vi "generate path.vi"(8 "Config":T1={"Path"={"Spacing"=2608.0, "Smooth Weight"=0.3, "Tolerance"=0.01}, "Kinematics"={"Max Vel"=2000.0, "Max Accel"=200.0, "Curvature Const"=2.0}}, 11 "Waypoints":dbl[][](array[numeric])=[[0.0, 0.0], [100.0, 15648.0], [10342.0, 25000.0]]) -> (0 "Target Velocities":dbl[](array[numeric])=[2000.0, 2000.0, 2000.0, 2000.0, 2000.0, 2000.0, 2000.0, 2000.0, 2000.0, 2000.0, 2000.0, 2000.0, 711.0227082060944, 0.0], 1 "Curvatures":dbl[](array[numeric])=[0.0, 3.4302286185049717e-08, 1.4910129056131163e-07, 6.219521538995594e-07, 2.6949817858486045e-06, 1.4154000940659975e-05, 0.00023495395525552563, 0.00023525971283188817, 1.4187548384027874e-05, 2.7111182211640585e-06, 6.348598719882183e-07, 1.6153870928568953e-07, 3.791514640017743e-08, 0.0], 2 "Distances":dbl[](array[numeric])=[0.0, 2607.53403486597, 5213.983232262121, 7815.725274588733, 10398.164925443389, 12901.736731112851, 15084.281319487234, 16023.34722695848, 18204.75324450246, 20703.52584101628, 23266.310669669037, 25787.681820994472, 28065.50969532439, 29329.39292428621], 3 "Smooth Path":dbl[][](array[numeric])=[[0.0, 0.0], [16.762978418693848, 2607.480152472678], [33.754054739996675, 5213.873968060124], [51.726604027530996, 7815.553933444405], [73.73097712533784, 10397.899835501465], [112.22196059188855, 12901.17573526458], [218.12358455167686, 15081.149525539358], [599.651678730881, 15939.217758214812], [2147.0337138764517, 17476.79411426541], [3977.030345252475, 19178.257254695087], [5865.836303317633, 20910.38834983492], [7726.868088266148, 22611.527138454912], [9408.73579474731, 24147.697976275413], [10342.0, 25000.0]], 4 "Max Velocities":dbl[](array[numeric])=[2000.0, 2000.0, 2000.0, 2000.0, 2000.0, 2000.0, 2000.0, 2000.0, 2000.0, 2000.0, 2000.0, 2000.0, 2000.0, 0.0], 5 "Path":dbl[][](array[numeric])=[[0.0, 0.0], [16.666326346427997, 2607.946746689072], [33.332652692855994, 5215.893493378144], [49.998979039283995, 7823.840240067216], [66.66530538571199, 10431.786986756288], [83.33163173213998, 13039.733733445359], [99.99795807856798, 15647.68048013443], [100.0, 15648.0], [2025.9131733642275, 17406.55692221268], [3951.826346728455, 19165.11384442536], [5877.739520092682, 20923.67076663804], [7803.65269345691, 22682.22768885072], [9729.565866821138, 24440.7846110634], [10342.0, 25000.0]])   [LabVIEW 2018]
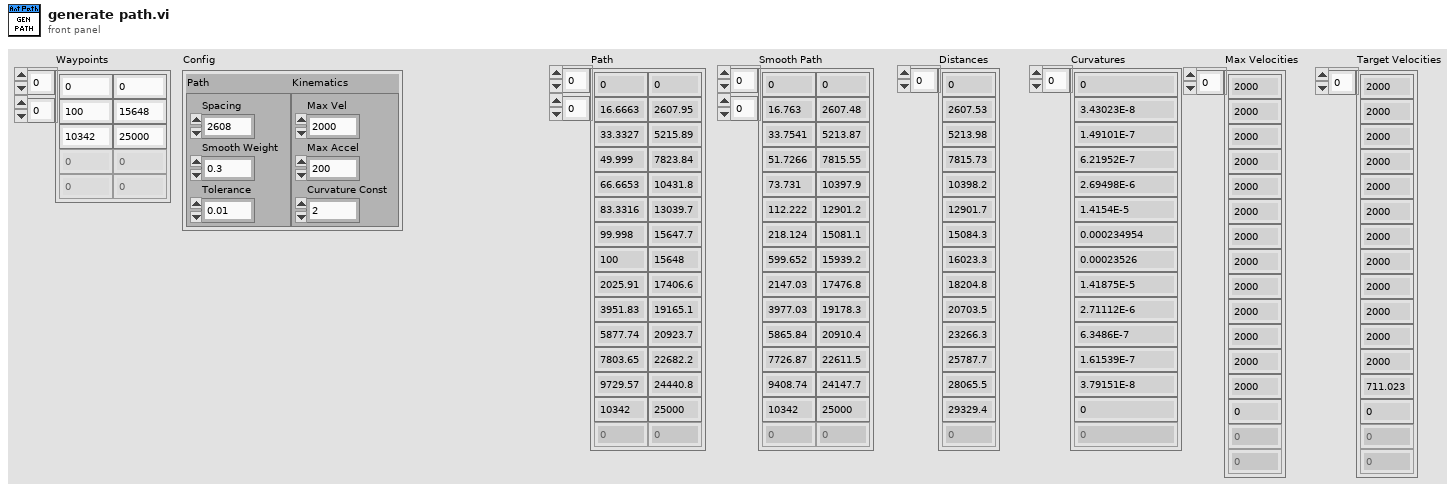
[diagram p1: front panel]
types:
  T1 = cluster{"Path":cluster{"Spacing":dbl, "Smooth Weight":dbl, "Tolerance":dbl}, "Kinematics":cluster{"Max Vel":dbl, "Max Accel":dbl, "Curvature Const":dbl}}
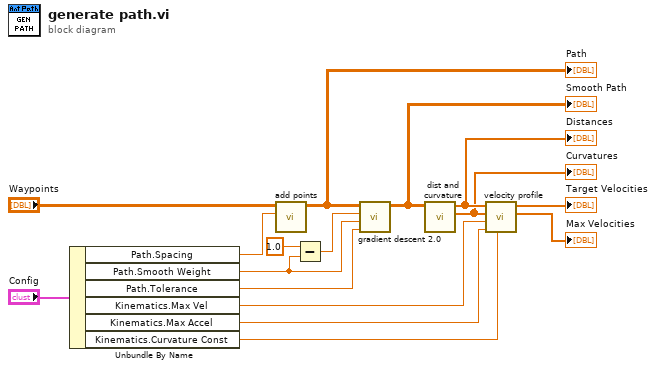
[diagram p0: block diagram]
diagram:
  n1 = Unbundle By Name("Config") -> ("Path.Spacing"=w8:dbl, "Path.Smooth Weight"=w14:dbl, "Path.Tolerance"=w13:dbl, "Kinematics.Max Vel"=w12:dbl, "Kinematics.Max Accel"=w11:dbl, "Kinematics.Curvature Const"=w10:dbl)
  n2 = call "add points.vi"("Spacing"=w8, "Waypoints"="Waypoints") -> ("Path"=w3:dbl[][])  [unwired: 9 in]
  "Path" <- w3
  n3 = Subtract(x=1.0, y=w14) -> (x-y=w15:dbl)
  n4 = call "gradient descent 2.0.vi"("tolerance"=w13, "weight_smooth"=w14, "weight_data"=w15, "Path"=w3) -> ("Smooth Path"=w2:dbl[][])  [unwired: 7 in]
  "Smooth Path" <- w2
  n5 = call "dist and curvature.vi"("Path"=w2) -> ("Curvatures"=w4:dbl[], "Distances"=w5:dbl[])  [unwired: 9 in]
  "Distances" <- w5
  "Curvatures" <- w4
  n6 = call "velocity profile.vi"("Konstant"=w10, "Max Accel"=w11, "Max Vel"=w12, "Curvatures"=w4, "Distances"=w5) -> ("Max Velocities"=→"Max Velocities":dbl[], "Target Velocities"=→"Target Velocities":dbl[])  [unwired: 5 in]
